vi "RP Lockin Proccess.vi"(4 "Save output":bool, 6 "CH index":i32, 7 "Internal configuration":T1={"Filter type"=enum."IIR", "Max points to plot"=100000, "X tiime shift"=0.0} {"X tiime shift" format="%#_6p"; "Max points to plot" format="%.5p"}, 8 "Error In":errorcluster, 10 "User configuration":T2={"Time constant"=0.0, "Phase"=0.0, "Signal channels"=[], "Group"="p", "X channel"="", "Live update"=TRUE} {"Phase" scale=-180.0..180.0; "Time constant" min=1e-06 max=1.0 scale=1e-06..0.01 scale format="%#_6p"}, 11 "Signal file":path) -> (0 "Error Out":errorcluster, 2 "XY Graph":cluster{dbl[], "Y":dbl[]}[](graph), 3 "Signal file out":path)   [LabVIEW 2016]
uses:
  <vilib>/Waveform/WDTOps.llb/WDT Get Waveform Time Array DBL.vi
  <vilib>/Waveform/WDTOps.llb/WDT Number of Waveform Samples DBL.vi
panel:
  out "Phase":dbl
  out "Waveform Graph 2":waveform(dbl)(graph)
  in  "Fix time delay":bool=TRUE
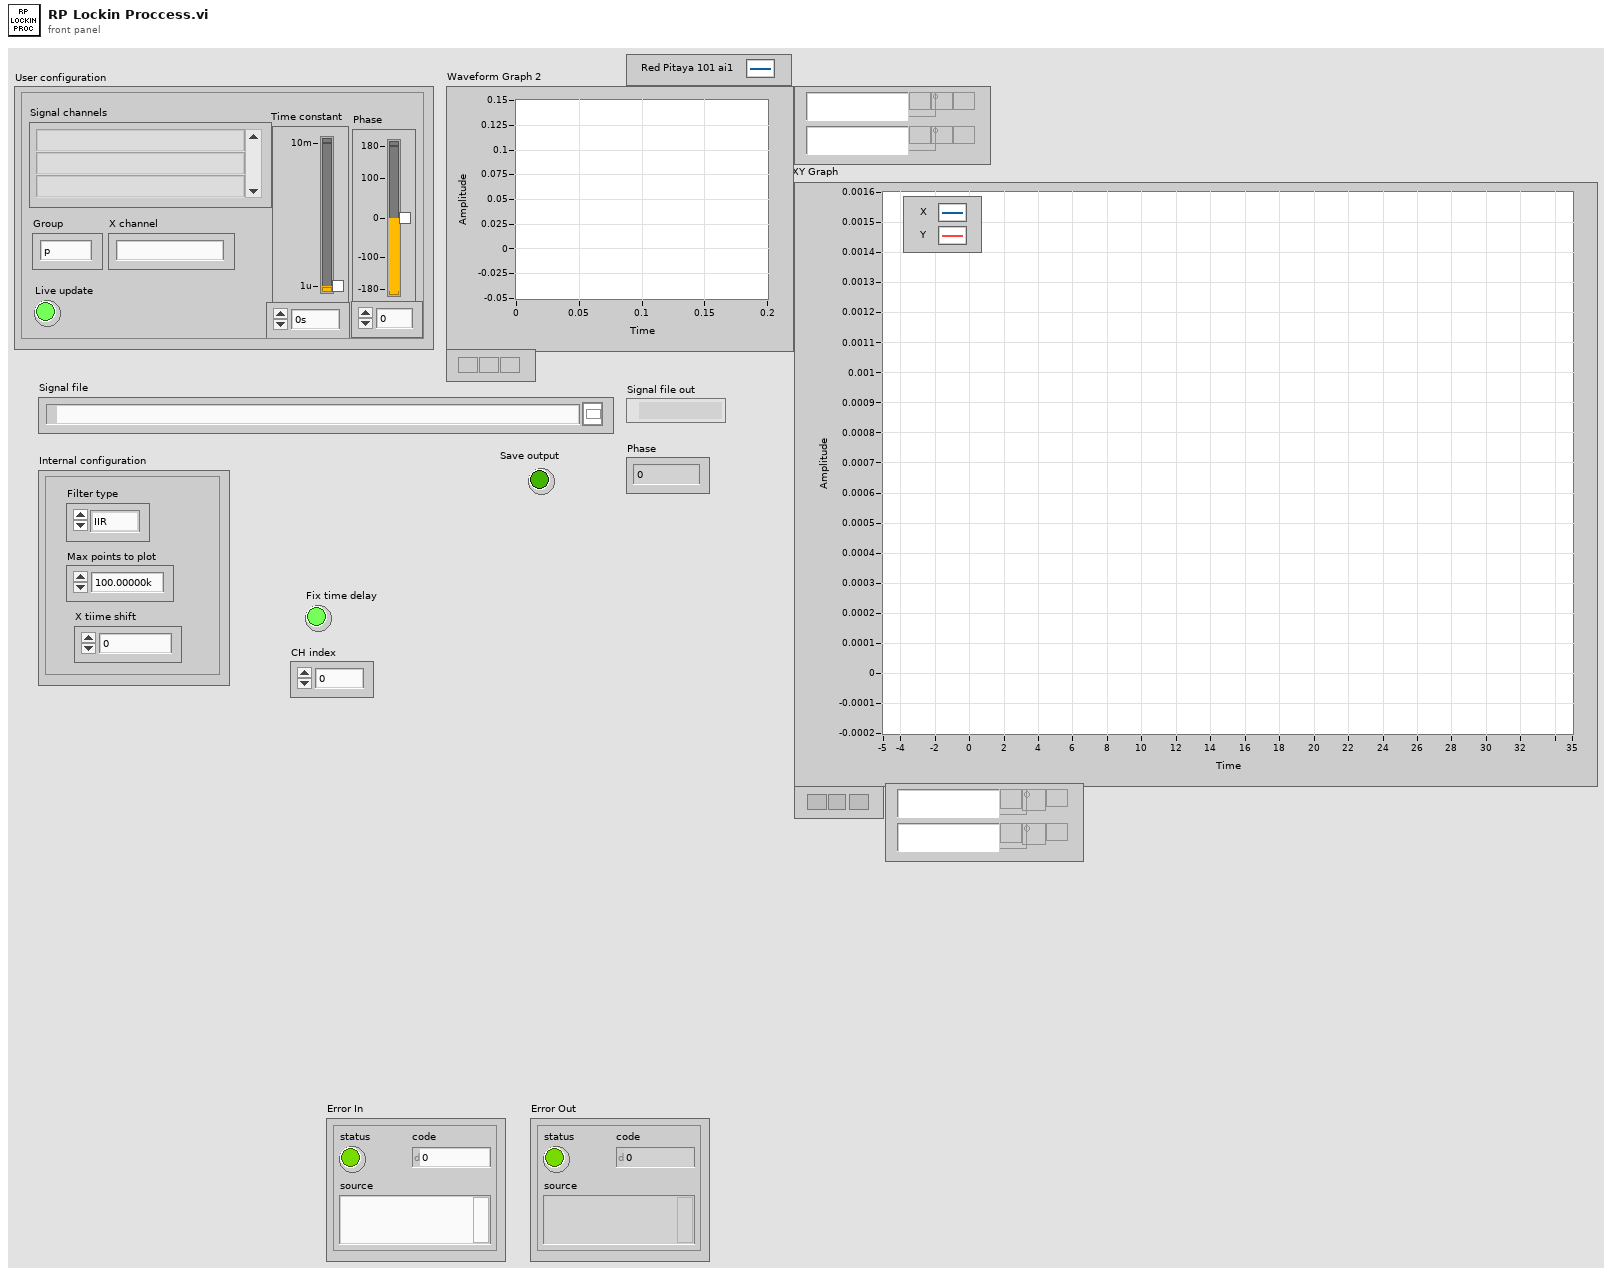
[diagram p1: front panel]
types:
  T1 = cluster{"Filter type":enum16{"None", "IIR", "FIR"}, "Max points to plot":i32, "X tiime shift":dbl}
  T2 = cluster{"Time constant":dbl, "Phase":dbl, "Signal channels":string[], "Group":string, "X channel":string, "Live update":bool}
  T3 = enum16{"open", "open or create", "create or replace", "create", "open (read-only)"}
  T4 = cluster{"Waveform":waveform(dbl), "Waveform":waveform(dbl)}
  T5 = cluster{"Waveform":waveform(dbl), "Waveform":waveform(dbl)}[]
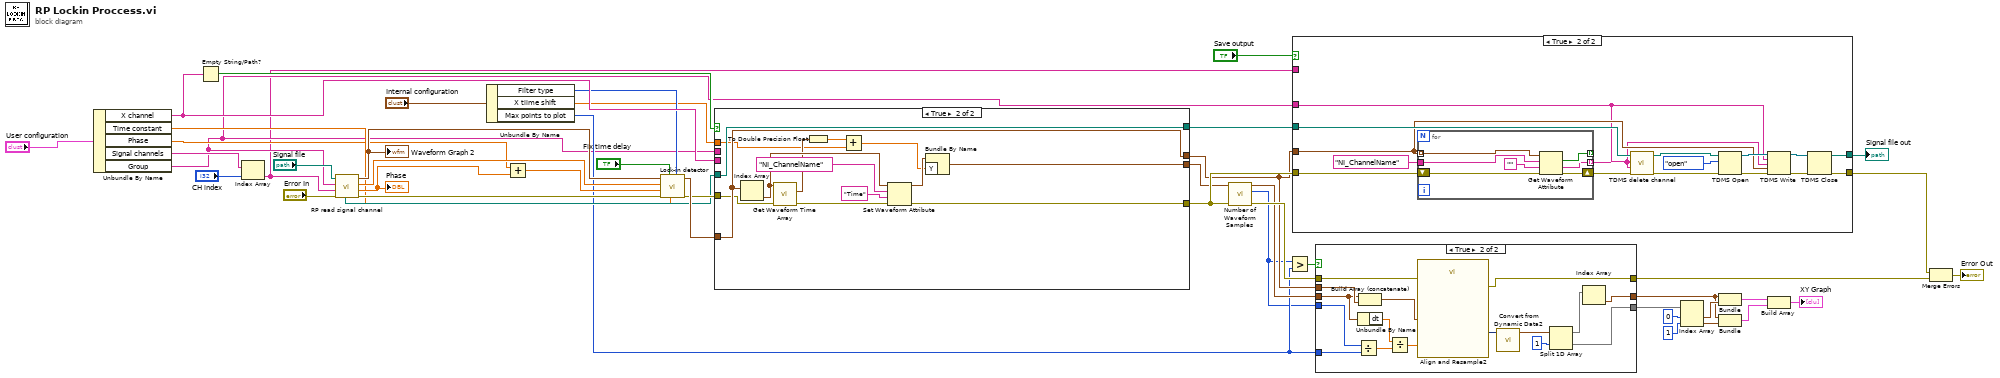
[diagram p0: block diagram]
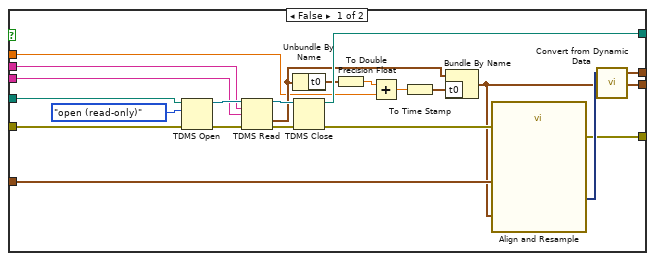
[diagram p3: hidden frame]
diagram:
  n1 = Unbundle By Name("User configuration") -> ("X channel"=w31:string, "Time constant"=w4:dbl, "Phase"=w3:dbl, "Signal channels"=w33:string[], "Group"=w2:string)
  n2 = Empty String/Path?(string/path=w31) -> (empty?=w35:bool)
  n3 = Index Array(array=w33, index="CH index") -> (element=w1:string)
  n4 = call "RP read signal channel.vi"("Error In"="Error In", "Channel name"=w1, "group name in"=w2, "File"="Signal file") -> ("Error Out"=w44:errorcluster, "Phase"=w45:dbl, "Frequency"=w46:dbl, "Data out"=w36:waveform(dbl), "File out"=w29:path)  [unwired: 1 in, 2 out]
  "Waveform Graph 2" <- w36
  "Phase" <- w45
  n5 = Unbundle By Name("Internal configuration") -> ("Filter type"=w27:enum16{"None", "IIR", "FIR"}, "X tiime shift"=w26:dbl, "Max points to plot"=w13:i32)
  n6 = Add(x=w3, y=w45) -> (x+y=w41:dbl)
  n7 = call "Lock-in detector.vi"("Filter type"=w27, "Time constant"=w4, "Fix time delay"="Fix time delay", "Error In"=w44, "Phase"=w41, "Frequency"=w46, "Data in"=w36) -> ("Error Out"=w37:errorcluster, "Data out"=w42:waveform(dbl)[])  [unwired: 3 in]
  n8 = case shown="True" w35 {
    tunnel: w42 -> [w63 w81]
    tunnel: [w61 w82] -> w39
    tunnel: [w48 w81] -> w14
    tunnel: w29 -> [w60 w82]
    tunnel: w37 -> [w57 w69]
    tunnel: [w58 w70] -> w17
    tunnel: w31 -> [w51 _]
    tunnel: w2 -> [w50 _]
    tunnel: w26 -> [w49 w72]
    tunnel: [w47 w71] -> w10
    frame False {
      n9 = TDMS Open(8:w57, 10:T3."open (read-only)" ("operation (0:open)"), 11:w60) -> (0:w67:errorcluster, 3:w66:refnum<k34>)  [unwired: 4 in]
      n10 = TDMS Read(0:w66, 5:w50, 7:w51, 11:w67) -> (4:w64:refnum<k34>, 10:w52:waveform(dbl), 15:w65:errorcluster)  [unwired: 4 in, 3 out]
      n11 = Unbundle By Name(w52) -> ("t0"=w56:timestamp)
      n12 = TDMS Close(8:w65, 11:w64) -> (0:w59:errorcluster, 3:w61:path)
      n13 = To Double Precision Float(number=w56) -> (double precision float=w55:dbl)
      n14 = Add(x=w55, y=w49) -> (x+y=w54:dbl)
      n15 = To Time Stamp(1:w54) -> (0:w53:timestamp)
      n16 = Bundle By Name(cluster=w52, "t0"=w53) -> (w47:waveform(dbl))
      n17 = call "Align and Resample"("Reference Signal"=w47, "error in (no error)"=w59, "Signals"=w63) -> ("error out"=w58:errorcluster, "Resampled Signals"=w62:dynamicdata)  [unwired: 6 in, 1 out]
      n18 = call "Convert from Dynamic Data"("Dynamic Data Type"=w62) -> ("Array of Waveform"=w48:waveform(dbl)[])  [unwired: 3 in]
    }
    frame True {
      n19 = Index Array(array=w81) -> (element=w77:waveform(dbl))  [unwired: 1 in]
      n20 = call-poly <vilib>:"Get Waveform Time Array.vi"("error in (no error)"=w69, "waveform in"=w77) -> ("error out"=w78:errorcluster, "X array"=w76:timestamp[])  [unwired: 8 in]
      n21 = To Double Precision Float(number=w76) -> (double precision float=w73:dbl[])
      n22 = Add(x=w73, y=w72) -> (x+y=w74:dbl[])
      n23 = Set Waveform Attribute(4:w78, 5:"Time", 6:"NI_ChannelName" ("name"), 7:w77) -> (0:w70:errorcluster, 3:w75:waveform(dbl))  [unwired: 1 out]
      n24 = Bundle By Name(cluster=w75, "Y"=w74) -> (w71:waveform(dbl))
    }
  }
  n25 = call-poly <vilib>:"Number of Waveform Samples.vi"("error in (no error)"=w17, "waveform in"=w10) -> ("error out"=w16:errorcluster, "number of samples"=w12:i32, "waveform out"=w15:waveform(dbl))  [unwired: 7 in]
  n26 = Greater?(x=w12, y=w13) -> (0:w18:bool)
  n27 = case shown="True" "Save output" {
    tunnel: w39 -> [w83 w96]
    tunnel: w17 -> [w84 w90]
    tunnel: [w84 w98] -> w38
    tunnel: w1 -> [_ _]
    tunnel: w14 -> [_ w88]
    tunnel: w2 -> [_ w87]
    tunnel: [w83 w85] -> w30
    frame False {
    }
    frame True {
      n28 = for {
        tunnel: w88 -> [w107] mode=indexing
        tunnel: "NI_ChannelName" ("name") -> [w106]
        tunnel: [w105] -> _ mode=indexing
        tunnel: [w101] -> w86 mode=indexing
        shift-right: [w103] -> w89
        shift-left: w90 -> [w104]
        n29 = Get Waveform Attribute(4:w104, 5:"", 6:w106, 7:w107) -> (0:w103:errorcluster, 1:w101:string, 2:w105:bool)  [unwired: 1 out]
      }
      n30 = call "TDMS delete channel.vi"("error in (no error)"=w89, "Channels"=w86, "group name"=w87, "file path"=w96) -> ("error out"=w95:errorcluster, "file path out"=w94:path)  [unwired: 5 in, 1 out]
      n31 = TDMS Open(8:w95, 10:T3."open" ("operation (0:open)"), 11:w94) -> (0:w92:errorcluster, 3:w93:refnum<k34>)  [unwired: 4 in]
      n32 = TDMS Write(0:w93, 5:w87, 7:w86, 9:w88, 11:w92) -> (4:w100:refnum<k34>, 15:w99:errorcluster)  [unwired: 1 in, 2 out]
      n33 = TDMS Close(8:w99, 11:w100) -> (0:w98:errorcluster, 3:w85:path)
    }
  }
  "Signal file out" <- w30
  n34 = case shown="True" w18 {
    tunnel: w16 -> [w108 w126]
    tunnel: w15 -> [w110 w123]
    tunnel: w14 -> [w109 w125]
    tunnel: w13 -> [_ w121]
    tunnel: w12 -> [_ w120]
    tunnel: [w108 w114] -> w7
    tunnel: [w109 w113] -> w11
    tunnel: [w110 w111] -> w9
    frame False {
    }
    frame True {
      n35 = Divide(x=w120, y=w121) -> (x/y=w119:dbl)
      n36 = Unbundle By Name(w123) -> ("dt"=w122:dbl)
      n37 = Build Array (concatenate)(w123, w125) -> (w124:waveform(dbl)[])
      n38 = Divide(x=w122, y=w119) -> (x/y=w118:dbl)
      n39 = call "Align and Resample2"("dt"=w118, "error in (no error)"=w126, "Signals"=w124) -> ("error out"=w114:errorcluster, "Resampled Signals"=w117:dynamicdata)  [unwired: 6 in, 1 out]
      n40 = call "Convert from Dynamic Data2"("Dynamic Data Type"=w117) -> ("Array of Waveform"=w116:waveform(dbl)[])  [unwired: 3 in]
      n41 = Split 1D Array(array=w116, index=1) -> (first subarray=w112:waveform(dbl)[], second subarray=w113:waveform(dbl)[])
      n42 = Index Array(array=w112) -> (element=w111:waveform(dbl))  [unwired: 1 in]
    }
  }
  n43 = Index Array(array=w11, index #1=0 ("index"), index #2=1 ("index")) -> (element #1=w22:waveform(dbl), element #2=w21:waveform(dbl))
  n44 = Bundle("Waveform"=w9, "Waveform"=w22) -> (w24:T4)  [unwired: 1 in]
  n45 = Bundle("Waveform"=w9, "Waveform"=w21) -> (w25:T4)  [unwired: 1 in]
  n46 = Build Array(w24, w25) -> (→"XY Graph":T5)
  n47 = Merge Errors(w38, w7) -> (→"Error Out":errorcluster)
